vi "GENser Revision Query.vi"(7 "GEN Addr":i16=-1, 8 "error":errorcluster, 11 "VISA":refnum<visa-resource-name>) -> (0 "error out":errorcluster, 1 "Driver Rev":string, 2 "Instrument Rev":string, 3 "VISA out":refnum<visa-resource-name>)   [LabVIEW 2017]
doc: "This VI queries the instrument firmware revision and instrument driver revision.\n\nInstrument Driver Name: LamGenPS.llb\nInstrument Manufacturer: Lambda\nInstrument Type: DC Power Supply\nSupported Models: Genesys Series\nSupported Bus Types: Serial: RS-232 or RS-485\n\nInstrument Driver Version: B03\nSupported Firmware: \"1.9\" and above\n\nCreated By: Walter Heyck\nRelease Date: July 2005\nOriginally Developed in LabVIEW Version: 6.1\nOriginally Developed using VISA Version: 3.1\n\nUnsupported Instrument Features: \n- SRQ interrupts \n- Event and Enable registers\n- Self-Test\n- Calibration commands\n\nModification History: \n\nREV_A00, Aug 2003\nInitial Release\n\nREV_B03, July 2005\nRewritten to follow \"Plug and Play\" driver standards, adds menu files for function pallet."
panel:
  # "Lambda Genesys \nSerial Port\n  DC Power Supplies"
  # "Read Revisions"
  # "-1 = no address change"
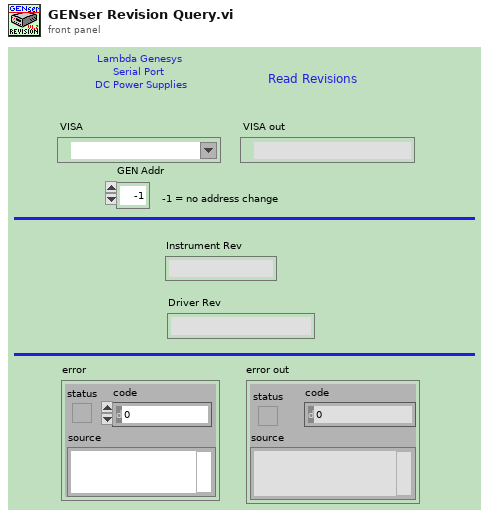
[diagram p1: front panel]
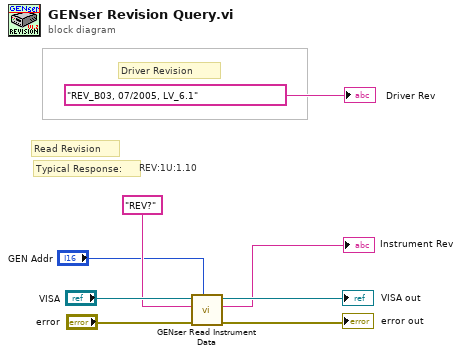
[diagram p0: block diagram]
diagram:
  # "REV:1U:1.10"
  # "Typical Response:"
  # "Driver Revision"
  # "Read Revision"
  n1 = call "GENser Read Instrument Data.vi"("GEN Addr"="GEN Addr", "error"="error", "Query"="REV?", "VISA"="VISA") -> ("error out"=→"error out":errorcluster, "Response"=→"Instrument Rev":string, "VISA out"=→"VISA out":refnum<visa-resource-name>)  [unwired: 4 in, 1 out]
  "Driver Rev" <- "REV_B03, 07/2005, LV_6.1" ("Instrument Driver Revision")
